vi "Read Sing.vi"(8 "error in (no error)":errorcluster, 11 "Peasant in":refnum<class "Peasant.lvclass">) -> (0 "error out":errorcluster, 2 "Sing":i32, 3 "Peasant out":refnum<class "Peasant.lvclass">)   [LabVIEW 2021]
uses:
  Peasant.lvclass
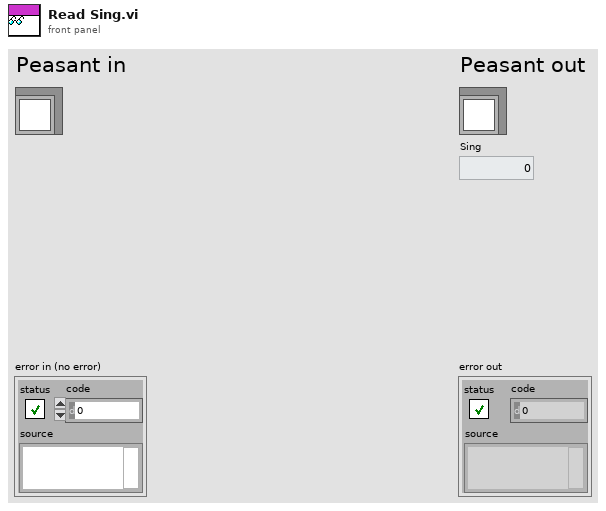
[diagram p1: front panel]
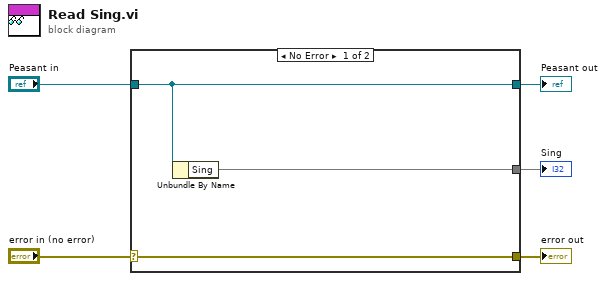
[diagram p0: block diagram]
diagram:
  n1 = case shown="No Error" "error in (no error)" {
    selector: "error in (no error)" -> [w8 w9]
    tunnel: [w8 w9] -> w4
    tunnel: [w7 w10] -> w2
    tunnel: "Peasant in" -> [w7 w10]
    tunnel: [w6 _] -> w1
    frame No Error {
      n2 = Unbundle By Name(w7) -> ("Sing"=w6)
    }
    frame Error {
    }
  }
  "error out" <- w4
  "Peasant out" <- w2
  "Sing" <- w1
